vi "Convert to Remote Instrument State.vi"(8 "error in (no error)":errorcluster, 11 "Internal Instrument State in":T2) -> (0 "error out":errorcluster, 3 "Remote Instrument State out":variant)   [LabVIEW 2020, in "Rename to match project.lvlib" / "Remote Connection Manager.lvlib"]
doc: "Converts the internal instrument state cluster into the remote instrument state representation."
uses:
  Remote Connection Manager.lvlib
  Instrument Manager/Instrument State.ctl
  Typedefs/Remote Instrument State.ctl
  Rename to match project.lvlib
  Instrument Manager/Instrument Manager.lvlib
panel:
  out "Remote Instrument State":T1
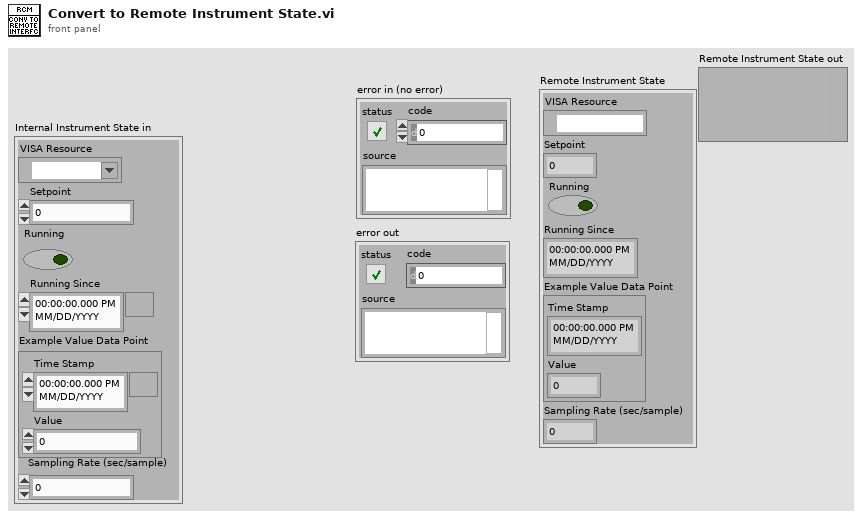
[diagram p1: front panel]
types:
  T1 = typedef "Rename to match project.lvlib/Remote Instrument State.ctl" = cluster{"VISA Resource":refnum<visa-resource-name>, "Setpoint":dbl, "Running":bool, "Running Since":timestamp, "Example Value Data Point":cluster{"Time Stamp":timestamp, "Value":dbl}, "Sampling Rate (sec/sample)":dbl}
  T2 = typedef "Rename to match project.lvlib/Instrument Manager.lvlib/Instrument State.ctl" = cluster{"VISA Resource":refnum<visa-resource-name>, "Setpoint":dbl, "Running":bool, "Running Since":timestamp, "Example Value Data Point":cluster{"Time Stamp":timestamp, "Value":dbl}, "Sampling Rate (sec/sample)":dbl}
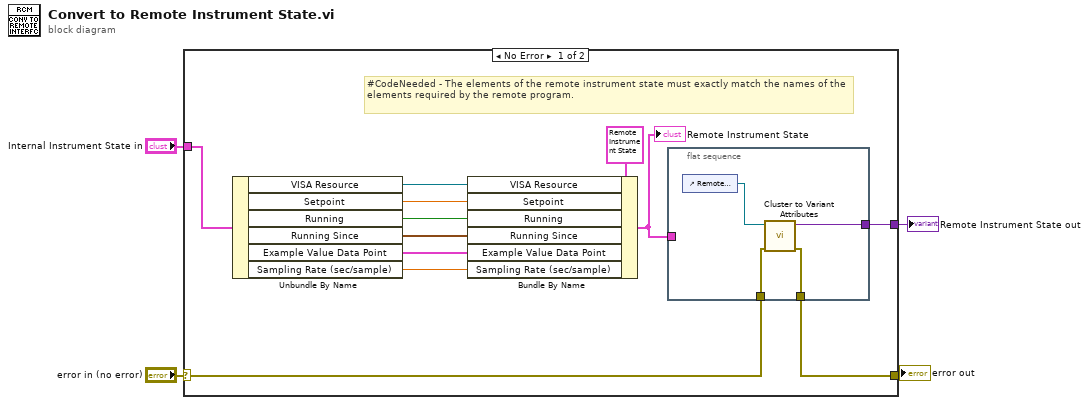
[diagram p0: block diagram]
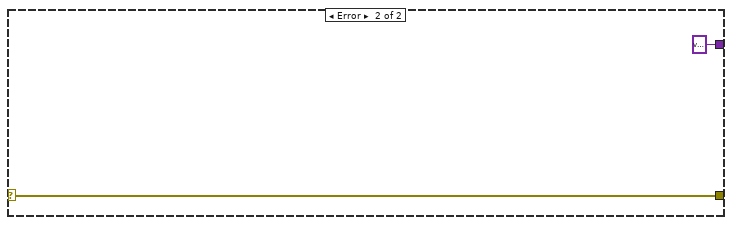
[diagram p2: hidden frame]
diagram:
  n1 = case shown="No Error" "error in (no error)" {
    selector: "error in (no error)" -> [w7 w22]
    tunnel: "Internal Instrument State in" -> [w16 _]
    tunnel: [w6 w22] -> w2
    tunnel: [w8 variant ("Variant out")] -> w1
    frame No Error {
      # "#CodeNeeded - The elements of the remote instrument state must exactly match the names of the elements required by the remote program."
      n2 = Unbundle By Name(w16) -> ("VISA Resource"=w14:refnum<visa-resource-name>, "Setpoint"=w13:dbl, "Running"=w12:bool, "Running Since"=w11:timestamp, "Example Value Data Point"=w10:cluster{"Time Stamp":timestamp, "Value":dbl}, "Sampling Rate (sec/sample)"=w9:dbl)
      n3 = Bundle By Name(cluster=T1 {"VISA Resource"="", "Setpoint"=0.0, "Running"=FALSE, "Running Since"=timestamp(0 s since 1904-01-01), "Example Value Data Point"={"Time Stamp"=timestamp(0 s since 1904-01-01), "Value"=0.0}, "Sampling Rate (sec/sample)"=0.0} ("Pump Controller State"), "VISA Resource"=w14, "Setpoint"=w13, "Running"=w12, "Running Since"=w11, "Example Value Data Point"=w10, "Sampling Rate (sec/sample)"=w9) -> (w5:T1)
      "Remote Instrument State" <- w5
      n4 = flat-sequence {
        tunnel: [w19] -> w8
        tunnel: w7 -> [w18]
        tunnel: [w17] -> w6
        tunnel: w5 -> [_]
        frame #0 {
          n5 = control-ref of="Remote Instrument State"() -> (w20:refnum<vi>)
          n6 = call "Cluster to Variant Attributes.vi"("error in (no error)"=w18, "Cluster in"=w20) -> ("error out"=w17:errorcluster, "Variant out"=w19:variant)  [unwired: 8 in]
        }
      }
    }
    frame Error {
    }
  }
  "error out" <- w2
  "Remote Instrument State out" <- w1
